vi "Auto Set Belt Speed.vi"(8 "error in":errorcluster, 9 "Auto Notifiers In":T1, 10 "Right Belt":dbl=1.0, 11 "Left Belt":dbl=1.0) -> (0 "error out":errorcluster, 1 "Auto Notifiers Out":T1)   [LabVIEW 2014]
doc: "Sets the Roller Speed"
uses:
  Auto Notifiers.ctl
  Main/Arms/Arm clapper state.ctl
  Main/Arms/Arm State.ctl
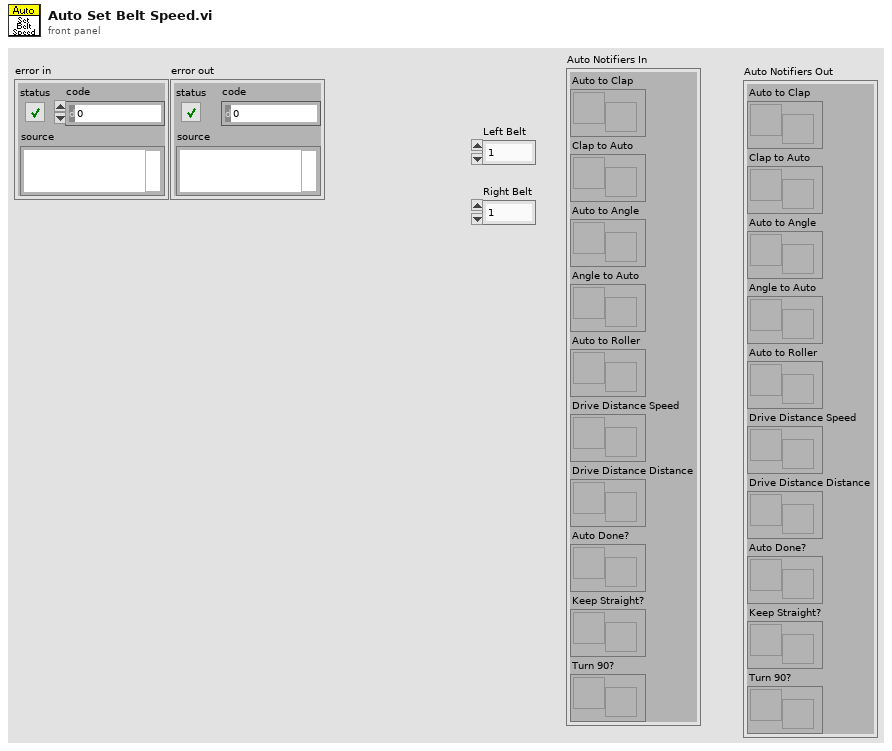
[diagram p1: front panel]
types:
  T1 = typedef "Auto Notifiers.ctl" = cluster{"Auto to Clap":refnum<notifier>, "Clap to Auto":refnum<notifier>, "Auto to Angle":refnum<notifier>, "Angle to Auto":refnum<notifier>, "Auto to Roller":refnum<notifier>, "Drive Distance Speed":refnum<notifier>, "Drive Distance Distance":refnum<notifier>, "Auto Done?":refnum<notifier>, "Keep Straight?":refnum<notifier>, "Turn 90?":refnum<notifier>}
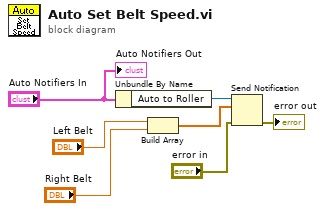
[diagram p0: block diagram]
diagram:
  n1 = Unbundle By Name("Auto Notifiers In") -> ("Auto to Roller"=w4:refnum<notifier>)
  n2 = Build Array("Left Belt", "Right Belt") -> (w5:dbl[])
  n3 = Send Notification(notification=w5, notifier=w4, error in (no error)="error in") -> (error out=→"error out":errorcluster)  [unwired: 1 out]
  "Auto Notifiers Out" <- "Auto Notifiers In"
